vi "DBL to String.vi"(7 "enable LabVIEW extensions?":bool, 11 "DBL":dbl) -> (3 "DBL string":string)   [LabVIEW 2017, in "JSONtext.lvlib"]
uses:
  JSONtext.lvlib
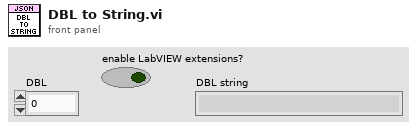
[diagram p1: front panel]
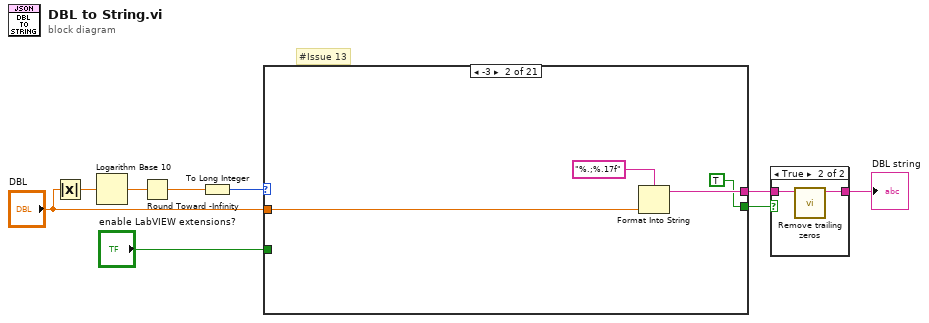
[diagram p0: block diagram]
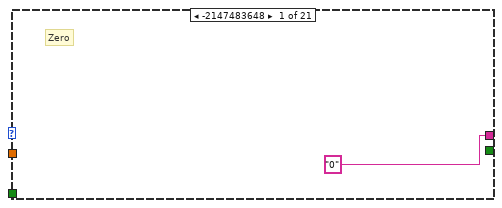
[diagram p3: hidden frame]
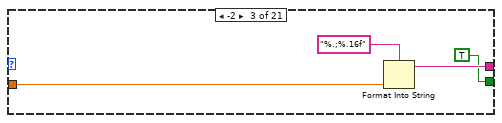
[diagram p4: hidden frame]
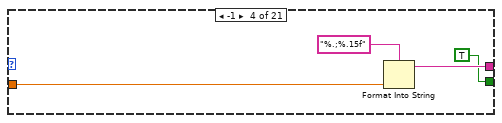
[diagram p5: hidden frame]
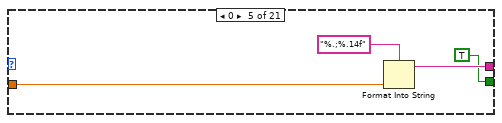
[diagram p6: hidden frame]
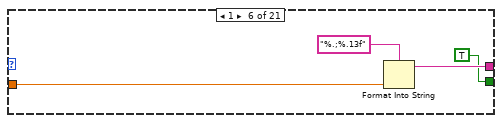
[diagram p7: hidden frame]
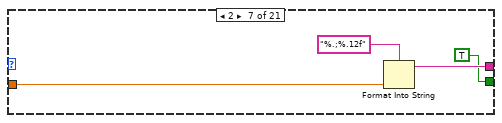
[diagram p8: hidden frame]
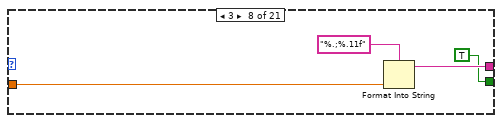
[diagram p9: hidden frame]
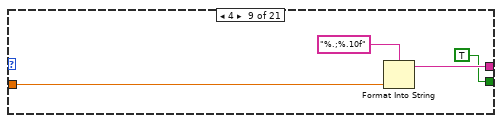
[diagram p10: hidden frame]
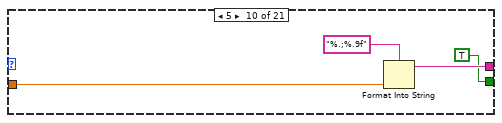
[diagram p11: hidden frame]
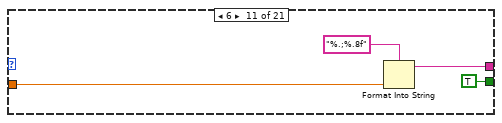
[diagram p12: hidden frame]
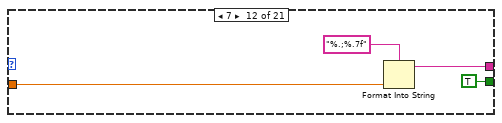
[diagram p13: hidden frame]
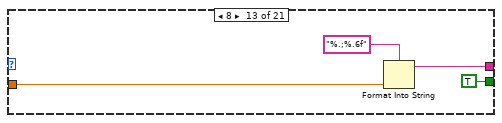
[diagram p14: hidden frame]
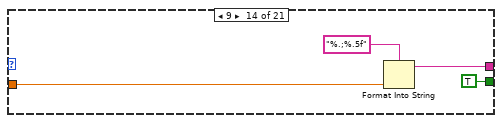
[diagram p15: hidden frame]
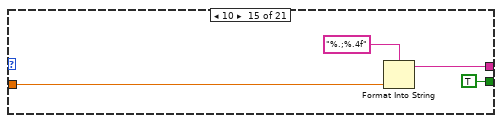
[diagram p16: hidden frame]
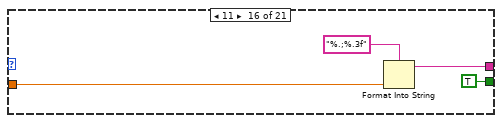
[diagram p17: hidden frame]
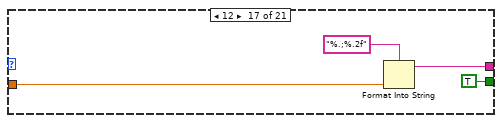
[diagram p18: hidden frame]
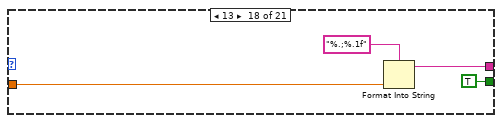
[diagram p19: hidden frame]
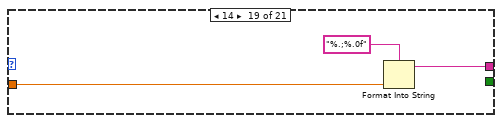
[diagram p20: hidden frame]
diagram:
  # "#Issue 13"
  n1 = Absolute Value(x="DBL") -> (abs(x)=w6:dbl)
  n2 = Logarithm Base 10(1:w6) -> (0:w3:dbl)
  n3 = Round Toward -Infinity(1:w3) -> (0:w4:dbl)
  n4 = To Long Integer(number=w4) -> (32bit integer=w5:i32)
  n5 = case shown="-3" w5 {
    tunnel: ["0" w14 w18 w22 w26 w30 w34 w38 w42 w46 w50 w54 w58 w62 w66 w70 w74 w78 w81 w82 w94] -> w8
    tunnel: "DBL" -> [_ w13 w17 w21 w25 w29 w33 w37 w41 w45 w49 w53 w57 w61 w65 w69 w73 w77 w80 w84 w95]
    tunnel: "enable LabVIEW extensions?" -> [_ _ _ _ _ _ _ _ _ _ _ _ _ _ _ _ _ _ _ w83 _]
    tunnel: [_ TRUE TRUE TRUE TRUE TRUE TRUE TRUE TRUE TRUE TRUE TRUE TRUE TRUE TRUE TRUE TRUE TRUE _ _ _] -> w9
    frame -2147483648 {
      # "Zero"
    }
    frame -3 {
      n6 = Format Into String(format string="%.;%.17f", w13) -> (resulting string=w14:string)  [unwired: 2 in, 1 out]
    }
    frame -2 {
      n7 = Format Into String(format string="%.;%.16f", w17) -> (resulting string=w18:string)  [unwired: 2 in, 1 out]
    }
    frame -1 {
      n8 = Format Into String(format string="%.;%.15f", w21) -> (resulting string=w22:string)  [unwired: 2 in, 1 out]
    }
    frame 0 {
      n9 = Format Into String(format string="%.;%.14f", w25) -> (resulting string=w26:string)  [unwired: 2 in, 1 out]
    }
    frame 1 {
      n10 = Format Into String(format string="%.;%.13f", w29) -> (resulting string=w30:string)  [unwired: 2 in, 1 out]
    }
    frame 2 {
      n11 = Format Into String(format string="%.;%.12f", w33) -> (resulting string=w34:string)  [unwired: 2 in, 1 out]
    }
    frame 3 {
      n12 = Format Into String(format string="%.;%.11f", w37) -> (resulting string=w38:string)  [unwired: 2 in, 1 out]
    }
    frame 4 {
      n13 = Format Into String(format string="%.;%.10f", w41) -> (resulting string=w42:string)  [unwired: 2 in, 1 out]
    }
    frame 5 {
      n14 = Format Into String(format string="%.;%.9f", w45) -> (resulting string=w46:string)  [unwired: 2 in, 1 out]
    }
    frame 6 {
      n15 = Format Into String(format string="%.;%.8f", w49) -> (resulting string=w50:string)  [unwired: 2 in, 1 out]
    }
    frame 7 {
      n16 = Format Into String(format string="%.;%.7f", w53) -> (resulting string=w54:string)  [unwired: 2 in, 1 out]
    }
    frame 8 {
      n17 = Format Into String(format string="%.;%.6f", w57) -> (resulting string=w58:string)  [unwired: 2 in, 1 out]
    }
    frame 9 {
      n18 = Format Into String(format string="%.;%.5f", w61) -> (resulting string=w62:string)  [unwired: 2 in, 1 out]
    }
    frame 10 {
      n19 = Format Into String(format string="%.;%.4f", w65) -> (resulting string=w66:string)  [unwired: 2 in, 1 out]
    }
    frame 11 {
      n20 = Format Into String(format string="%.;%.3f", w69) -> (resulting string=w70:string)  [unwired: 2 in, 1 out]
    }
    frame 12 {
      n21 = Format Into String(format string="%.;%.2f", w73) -> (resulting string=w74:string)  [unwired: 2 in, 1 out]
    }
    frame 13 {
      n22 = Format Into String(format string="%.;%.1f", w77) -> (resulting string=w78:string)  [unwired: 2 in, 1 out]
    }
    frame 14 {
      n23 = Format Into String(format string="%.;%.0f", w80) -> (resulting string=w81:string)  [unwired: 2 in, 1 out]
    }
    frame 2147483647 {
      n24 = case shown="True" w83 {
        tunnel: w84 -> [_ w87]
        tunnel: ["null" w86] -> w82
        frame False {
        }
        frame True {
          # "Inf OR -Inf or NaN"
          n25 = Format Into String(w87) -> (resulting string=w88:string)  [unwired: 3 in, 1 out]
          n26 = case shown="\"-Inf\"" w88 {
            tunnel: ["-Infinity" "NaN" "null" "Infinity"] -> w86
            frame "-Inf" {
            }
            frame "NaN" {
            }
            frame Default {
            }
            frame "Inf" {
            }
          }
        }
      }
    }
    frame Default {
      n27 = Format Into String(format string="%.;%.14e", w95) -> (resulting string=w94:string)  [unwired: 2 in, 1 out]
    }
  }
  n28 = case shown="True" w9 {
    tunnel: [w96 w98] -> w7
    tunnel: w8 -> [w96 w97]
    frame False {
    }
    frame True {
      n29 = call "Remove trailing zeros.vi"("Number"=w97) -> ("Number with trainlg zeros removed"=w98:string)  [unwired: 10 in]
    }
  }
  "DBL string" <- w7
